vi "Init Obj From Cnfg File.vi"(8 "error in (no error)":errorcluster, 10 "Card Config":T1={"Logical Name"="", "Base Settings"={"Clock Source"=1, " clock modulo"=1000000, "TriggerEnabled?"=TRUE, "trigger modulo "=0, "InputTerminated?"=FALSE, "Inhibit(µs)"=1.0, "TriggerLevel"=1.0, "PresetValue"=0, "InternalTrigger?"=FALSE, "InternalArm?"=FALSE, "SWTrigger?"=FALSE, "RisingEdge?"=FALSE, "StopOnPreset?"=FALSE, "ResetWhenDone?"=TRUE, "Gate Divider"=1, "PositiveGate?"=TRUE}, "SG08_Settings"={"Gate Terminate"=TRUE, "Gate Level"=1.0, "Gate Delay (µs)"=0.0, "StepBackTime (µs)"=0.0, "Burst Counter"=0, "Trigger Divider"=1, "Trigger Multiplier"=4}, "Channel Names"=[], "Advanced Settings"={"Trigger on MS Bus"=24, "Force Trigger (µs)"=0.0, "Gate Type"=TRUE, "Synchronize Gate"=FALSE}} {"Advanced Settings"."Trigger on MS Bus" format="%04x" items=["Local Primary0x1"=1, "Local Secondary0x2"=2, "Local Force 0x4"=4, "Resynchronize 0x8"=8, "StepBackOnBus 0x10"=16, "StartOnBus 0x20"=32, "InhibitOnBus 0x40"=64, "LoadDataOnBus 0x80"=128]; "Advanced Settings"."Force Trigger (µs)" min=0.0 format="%.6f"; "SG08_Settings"."StepBackTime (µs)" min=0.0 format="%.6f"; "SG08_Settings"."Gate Delay (µs)" format="%.3f"; "SG08_Settings"."Gate Level" min=-2.5 max=2.5 format="%.3g"; "Base Settings"."Gate Divider" min=1 max=1000000; "Base Settings"."Clock Source" items=["Internal Oscillator"=1, "External Trigger"=2, "Trigger-> Oscillator"=3, "MasterSlave Bus"=4]; "Base Settings"."Inhibit(µs)" format="%#_11g"}, 11 "BME_DG_G08 in":refnum<class "BME_DG_G08.lvclass">) -> (0 "error out":errorcluster, 3 "BME_DG_G08 out":refnum<class "BME_DG_G08.lvclass">)   [LabVIEW 2009, in "POLARIS BME DG.lvlib" / "BME_DG_G08.lvclass"]
uses:
  BME_DG_G08.lvclass
  Card Config.ctl
  LV-BME Interface/BME_DG_TriggerSettings.ctl
  LV-BME Interface/ClockSource.ctl
  SG08_Settings.ctl
  LV-BME Interface/BME_DG_V2TriggerSettings.ctl
  MSBusSignals.ctl
  BME_DG_G05P2/BME_DG_G05P2.lvclass
  POLARIS BME DG.lvlib
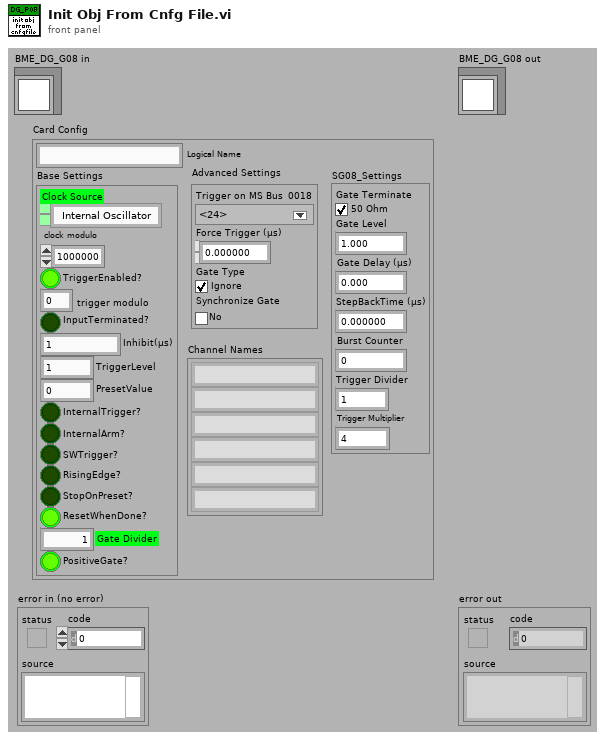
[diagram p1: front panel]
types:
  T1 = typedef "POLARIS BME DG.lvlib/Card Config.ctl" = cluster{"Logical Name":string, "Base Settings":T2, "SG08_Settings":T4, "Channel Names":string[], "Advanced Settings":T5}
  T2 = typedef "POLARIS BME DG.lvlib/BME_DG_TriggerSettings.ctl" = cluster{"Clock Source":T3, " clock modulo":u32, "TriggerEnabled?":bool, "trigger modulo ":i32, "InputTerminated?":bool, "Inhibit(µs)":dbl, "TriggerLevel":dbl, "PresetValue":i32, "InternalTrigger?":bool, "InternalArm?":bool, "SWTrigger?":bool, "RisingEdge?":bool, "StopOnPreset?":bool, "ResetWhenDone?":bool, "Gate Divider":i32, "PositiveGate?":bool}
  T3 = typedef "POLARIS BME DG.lvlib/ClockSource.ctl" = i32
  T4 = typedef "POLARIS BME DG.lvlib/SG08_Settings.ctl" = cluster{"Gate Terminate":bool, "Gate Level":dbl, "Gate Delay (µs)":dbl, "StepBackTime (µs)":dbl, "Burst Counter":u32, "Trigger Divider":u32, "Trigger Multiplier":u32}
  T5 = typedef "POLARIS BME DG.lvlib/BME_DG_V2TriggerSettings.ctl" = cluster{"Trigger on MS Bus":T6, "Force Trigger (µs)":dbl, "Gate Type":bool, "Synchronize Gate":bool}
  T6 = typedef "POLARIS BME DG.lvlib/MSBusSignals.ctl" = u32
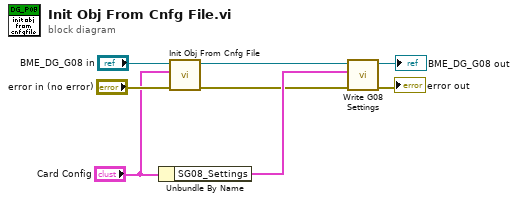
[diagram p0: block diagram]
diagram:
  n1 = Unbundle By Name("Card Config") -> ("SG08_Settings"=w5:T4)
  n2 = call-parent "Init Obj From Cnfg File.vi"("error in (no error)"="error in (no error)", "Card Config"="Card Config", "BME_DG_G05 in"="BME_DG_G08 in") -> ("error out"=w3:errorcluster, "BME_DG_G05 out"=w4:refnum<class "BME_DG_G08.lvclass">)  [unwired: 7 in]
  n3 = call-dynamic "Write G08 Settings.vi"("error in (no error)"=w3, "SG08_Settings"=w5, "BME_DG_G08 in"=w4) -> ("error out"=→"error out":errorcluster, "BME_DG_G08 out"=→"BME_DG_G08 out":refnum<class "BME_DG_G08.lvclass">)  [unwired: 7 in]
